vi "File Analysis.vi"() -> ()   [LabVIEW 2025]
panel:
  in  "Y-AXIS":u16(ring) items=["None", "Time ( Sec )", "Normal Load ( N )", "Frictional Force ( N )", "Coefficient of Friction", "Depth ( Microns )", "Speed ( RPM )", "Frequency ( Hz )", "Angle ( Degree )", "Cyclic Friction Force ( N )", "Cyclic Co efficient Friction ", "Stage temperature ( Degree celcius )", "Sample temperature ( Degree celcius )", "Stroke Length ( mm )", "Scratch Speed ( mm/sec )", "Amb Humidity ( % Rh ) ", "Amb Temperature (Deg C)", "Acoustic (mV)", "Mx (Nm)", "My (Nm)", "Mz (Nm)", "Humidity ( % Rh )", "Sliding Distance (mm)", "Wear Track Diameter (mm)", "Fx(N)", "Fy(N)", "MTM BallSpeed (RPM)", "MTM DiscSpeed (RPM)", "Entrainment Speed", "Slide Role", "Slip(%)", "Rotary Speed (m/sec)", "MTM Ball Speed (m/sec)", "MTM Disc Speed (m/sec)", "ECR (ohms)"]
  in  "X-AXIS":u16(ring) items=["None", "Time ( Sec )", "Normal Load ( N )", "Frictional Force ( N )", "Coefficient of Friction", "Depth ( Microns )", "Speed ( RPM )", "Frequency ( Hz )", "Angle ( Degree )", "Cyclic Friction Force ( N )", "Cyclic Co efficient Friction ", "Stage temperature ( Degree celcius )", "Sample temperature ( Degree celcius )", "Stroke Length ( mm )", "Scratch Speed ( mm/sec )", "Amb Humidity ( % Rh ) ", "Amb Temperature (Deg C)", "Acoustic (mV)", "Mx (Nm)", "My (Nm)", "Mz (Nm)", "Humidity ( % Rh )", "Sliding Distance (mm)", "Wear Track Diameter (mm)", "Fx(N)", "Fy(N)", "MTM BallSpeed (RPM)", "MTM DiscSpeed (RPM)", "Entrainment Speed", "Slide Role", "Slip(%)", "Rotary Speed (m/sec)", "MTM Ball Speed (m/sec)", "MTM Disc Speed (m/sec)", "ECR (ohms)"]
  out "XY Graph":cluster{"Array 2":dbl[], "Array 2":dbl[]}[](graph) caption="XY Graph 20"
  in  "Analysis Home":bool
  out "File Name 2":string
  out "File Name 1":string
  in  "OPEN 2":bool
  in  "OPEN 1":bool
  in  "Refresh 2":bool
  out "File 1 Discription":string="\r"
  out "File 2 Discription":string="\r"
  out "File 3 Discription":string="\r"
  out "File 4 Discription":string="\r"
  in  "OPEN 4":bool
  out "File Name 4":string
  out "File Name 3":string
  in  "OPEN 3":bool
  out "MEAN":dbl format="%.3f"
  out "SD":dbl=-0.0 format="%.3f"
  out "VARIANCE":dbl=-0.0 format="%0.2f"
  out "MEAN 2":dbl format="%.3f"
  out "SD  2":dbl=-0.0 format="%.3f"
  out "VARIANCE 2":dbl=-0.0 format="%0.2f"
  out "MEAN  3":dbl format="%.3f"
  out "SD  3":dbl=-0.0 format="%.3f"
  out "VARIANCE  3":dbl=-0.0 format="%0.2f"
  out "MEAN 4":dbl format="%.3f"
  out "SD 4":dbl=-0.0 format="%.3f"
  out "VARIANCE 4":dbl=-0.0 format="%0.2f"
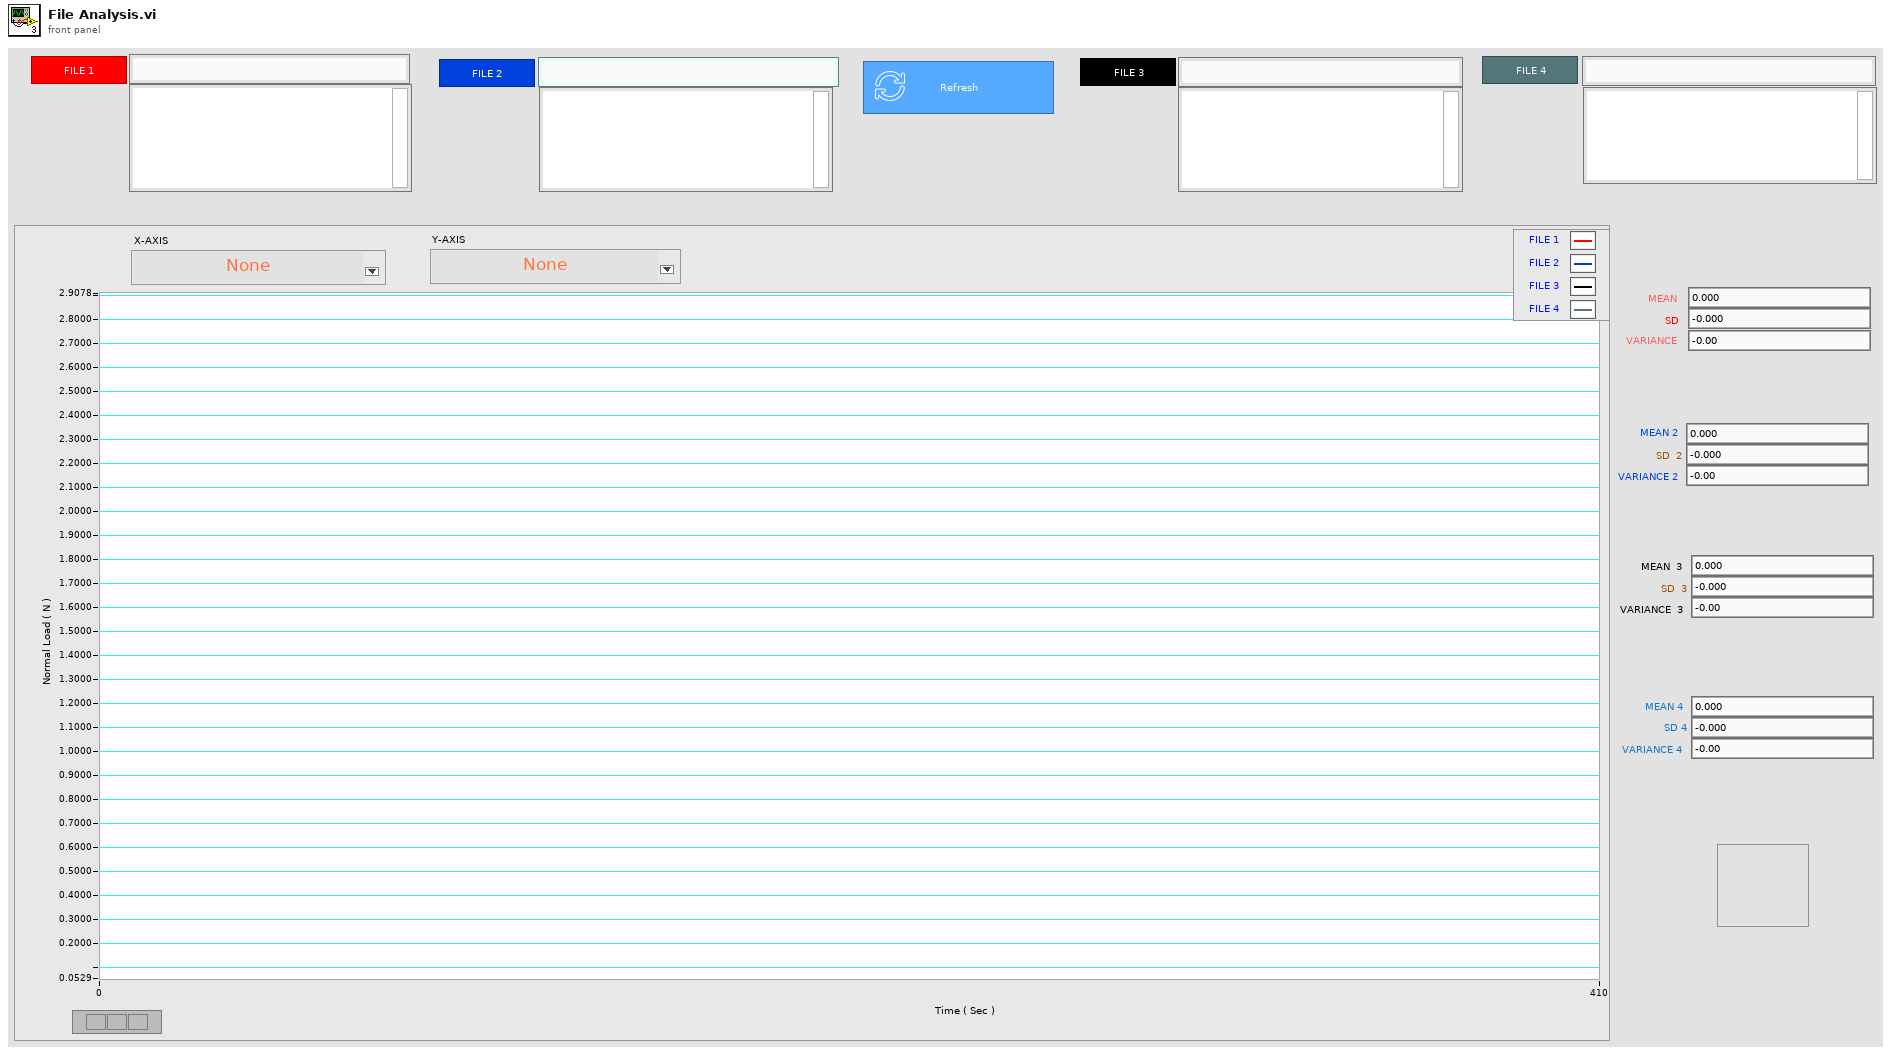
[diagram p1: front panel]
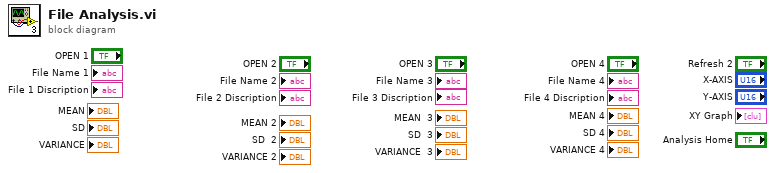
[diagram p0: block diagram]
diagram:
